vi "Calculate Vertex Array.vi"(8 "error in (no error)":errorcluster, 9 "Coordinates System":enum16{"Cartesian", "Cylindrical", "Spherical"}(ring)=enum."Spherical", 10 "3D Bar Datatype.lvclass in":refnum<class "3D Bar Datatype.lvclass">, 11 "Plot Representation In":T1) -> (0 "error out":errorcluster, 1 "Dup Coordinates System":enum16{"Cartesian", "Cylindrical", "Spherical"}(ring)=enum."Spherical", 2 "3D Bar Datatype.lvclass out":refnum<class "3D Bar Datatype.lvclass">, 3 "Plot Representation Out":T1)   [LabVIEW 2020, in "3D Bar Datatype.lvclass"]
uses:
  <vilib>/Math Plots/3D Math Plots/3D Bar/3D Bar Datatype/3D Bar Datatype.lvclass
  <vilib>/Math Plots/3D Math Plots/3D Plot/3D Plot/Typedef/Plot Representation.ctl
  <vilib>/Math Plots/3D Math Plots/3D Plot/3D Plot/Typedef/Range Clusters.ctl
  <vilib>/Math Plots/3D Math Plots/3D Plot/3D Plot/Typedef/Mesh Data.ctl
  <vilib>/Math Plots/3D Math Plots/3D Bar/3D Bar Datatype/3D Bar Datatype.lvclass/3D Bar Datatype.ctl
  <vilib>/Math Plots/3D Math Plots/3D Plot/3D Plot/3D Plot.lvclass
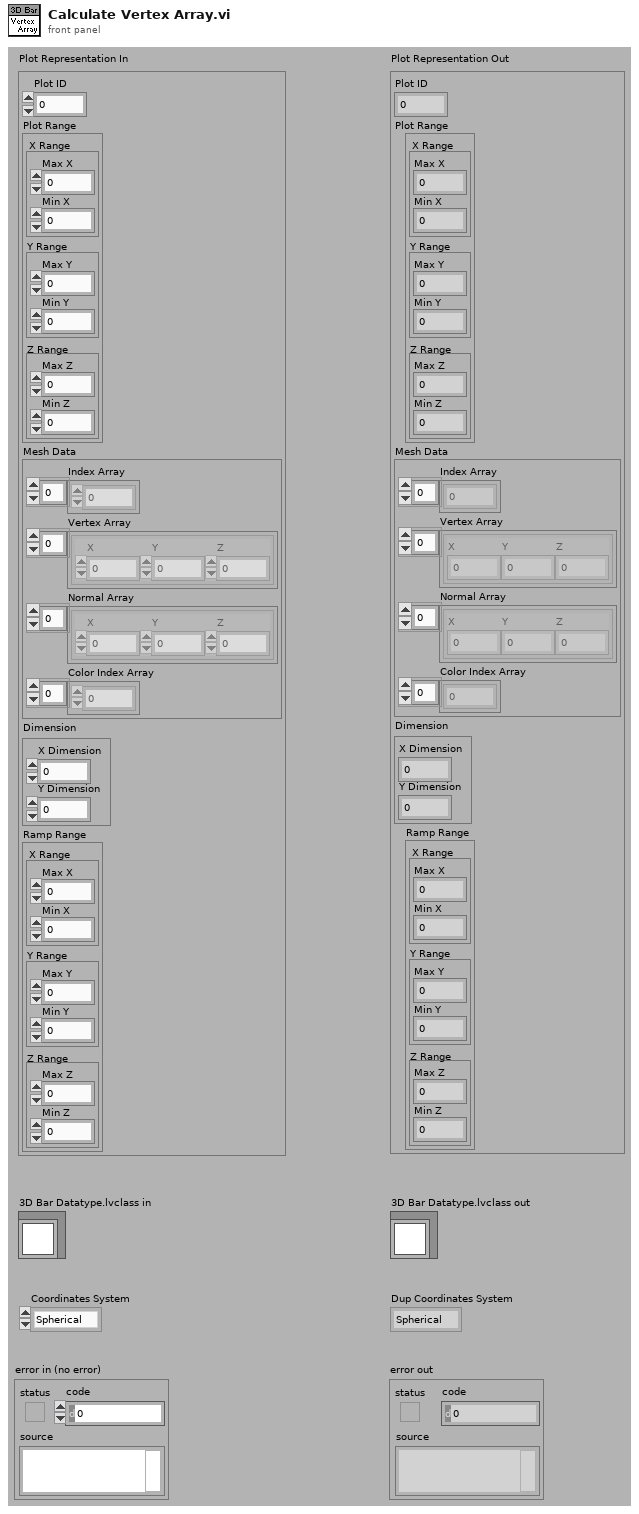
[diagram p1: front panel]
types:
  T1 = typedef "3D Plot.lvclass/Plot Representation.ctl" = cluster{"Plot ID":i32, "Plot Range":T2, "Mesh Data":T3, "Dimension":cluster{"X Dimension":i32, "Y Dimension":i32}, "Ramp Range":T2}
  T2 = typedef "3D Plot.lvclass/Range Clusters.ctl" = cluster{"X Range":cluster{"Max X":sgl, "Min X":sgl}, "Y Range":cluster{"Max Y":sgl, "Min Y":sgl}, "Z Range":cluster{"Max Z":sgl, "Min Z":sgl}}
  T3 = typedef "3D Plot.lvclass/Mesh Data.ctl" = cluster{"Index Array":u32[], "Vertex Array":cluster{"X":sgl, "Y":sgl, "Z":sgl}[], "Normal Array":cluster{"X":sgl, "Y":sgl, "Z":sgl}[], "Color Index Array":i32[]}
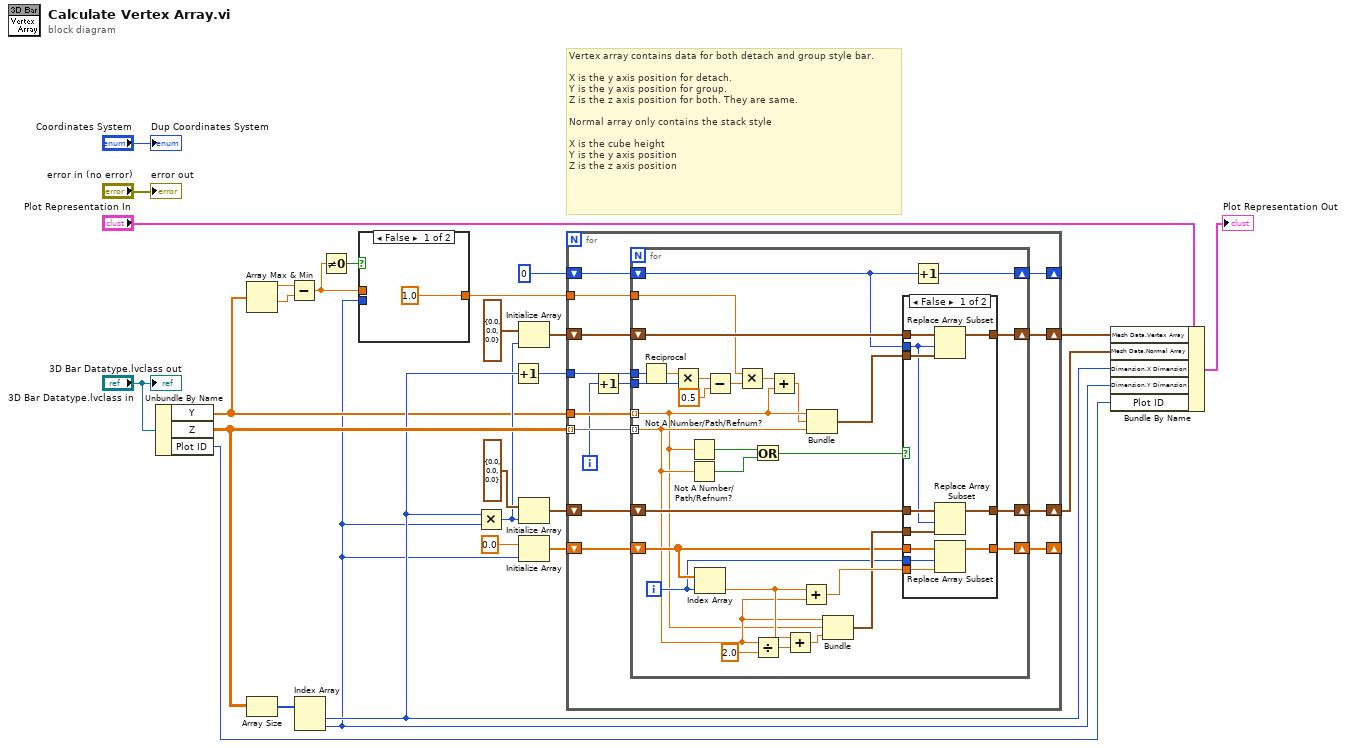
[diagram p0: block diagram]
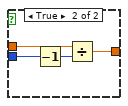
[diagram p2: hidden frame]
diagram:
  # "Vertex array contains data for both detach and group style bar. \n\nX is the y axis position for detach.\nY is the y axis position for group.\nZ is the z axis position for both. They are same.\n\nNormal array only contains the stack style\n\nX is the cube height\nY is the y axis position\nZ is the z axis position"
  n1 = Unbundle By Name("3D Bar Datatype.lvclass in") -> ("Y"=w7:sgl[], "Z"=w20:sgl[][], "Plot ID"=w19:i32)
  n2 = Array Max & Min(array=w7) -> (max value=w4:sgl, min value=w3:sgl)  [unwired: 2 out]
  n3 = Array Size(array=w20) -> (size(s)=w18:i32[])
  n4 = Subtract(x=w4, y=w3) -> (x-y=w2:sgl)
  n5 = Index Array(array=w18) -> (element #1=w15:i32, element #2=w5:i32)  [unwired: 2 in]
  n6 = Not Equal To 0?(x=w2) -> (x != 0?=w1:bool)
  n7 = case shown="False" w1 {
    tunnel: [sgl 1.0 w32] -> w6
    tunnel: w5 -> [_ w31]
    tunnel: w2 -> [_ w29]
    frame False {
    }
    frame True {
      n8 = Decrement(x=w31) -> (x-1=w30:i32)
      n9 = Divide(x=w29, y=w30) -> (x/y=w32:sgl)
    }
  }
  n10 = Multiply(x=w15, y=w5) -> (x*y=w11:i32)
  n11 = Increment(x=w15) -> (x+1=w21:i32)
  n12 = Initialize Array(cluster{"X":sgl, "Y":sgl, "Z":sgl} {"X"=0.0, "Y"=0.0, "Z"=0.0} ("3D Point"), w11) -> (w16:cluster{"X":sgl, "Y":sgl, "Z":sgl}[])
  n13 = Initialize Array(cluster{"X":sgl, "Y":sgl, "Z":sgl} {"X"=0.0, "Y"=0.0, "Z"=0.0} ("3D Point"), w11) -> (w10:cluster{"X":sgl, "Y":sgl, "Z":sgl}[])
  n14 = Initialize Array(sgl 0.0 ("y"), w5) -> (w9:sgl[])
  n15 = for {
    shift-right: [w45] -> w22
    shift-left: w16 -> [w46]
    tunnel: w20 -> [w44] mode=indexing
    tunnel: w7 -> [w43]
    tunnel: w21 -> [w42]
    shift-right: [w38] -> _
    shift-left: 0 -> [w39]
    shift-right: [w36] -> w8
    shift-left: w10 -> [w37]
    shift-right: [w34] -> _
    shift-left: w9 -> [w35]
    tunnel: w6 -> [w33]
    i -> [w41]
    n16 = Increment(x=w41) -> (x+1=w40:i32)
    n17 = for {
      shift-right: [w75] -> w45
      shift-left: w46 -> [w76]
      tunnel: w44 -> [w59] mode=indexing
      tunnel: w43 -> [w51] mode=indexing
      tunnel: w42 -> [w72]
      tunnel: w40 -> [w54]
      shift-right: [w73] -> w38
      shift-left: w39 -> [w63]
      shift-right: [w64] -> w36
      shift-left: w37 -> [w65]
      shift-right: [w61] -> w34
      shift-left: w35 -> [w62]
      tunnel: w33 -> [w48]
      i -> [w60]
      n18 = Reciprocal(x=w72) -> (1/x=w55:sgl)
      n19 = Multiply(x=w55, y=w54) -> (x*y=w53:sgl)
      n20 = Not A Number/Path/Refnum?(number/path/refnum=w51) -> (NaN/Path/Refnum?=w70:bool)
      n21 = Not A Number/Path/Refnum?(number/path/refnum=w59) -> (NaN/Path/Refnum?=w71:bool)
      n22 = Index Array(array=w62, index=w60) -> (element=w68:sgl)
      n23 = Subtract(x=w53, y=sgl 0.5) -> (x-y=w49:sgl)
      n24 = Multiply(x=w48, y=w49) -> (x*y=w47:sgl)
      n25 = Or(x=w70, y=w71) -> (x .or. y?=w56:bool)
      n26 = Divide(x=w59, y=sgl 2.0) -> (x/y=w58:sgl)
      n27 = Add(x=w47, y=w51) -> (x+y=w50:sgl)
      n28 = Add(x=w68, y=w58) -> (x+y=w67:sgl)
      n29 = Add(x=w68, y=w59) -> (x+y=w69:sgl)
      n30 = Bundle("Data"=w51, w50, "Data"=w59) -> (w74:cluster{"Data":sgl, sgl, "Data":sgl})  [unwired: 1 out]
      n31 = Bundle("Data"=w59, "Data"=w51, w67) -> (w66:cluster{"Data":sgl, "Data":sgl, sgl})  [unwired: 1 out]
      n32 = case shown="False" w56 {
        tunnel: w76 -> [w87 w90]
        tunnel: [w86 w90] -> w75
        tunnel: w74 -> [w85 _]
        tunnel: w69 -> [w84 _]
        tunnel: w66 -> [w83 _]
        tunnel: w65 -> [w82 w89]
        tunnel: [w81 w89] -> w64
        tunnel: w63 -> [w80 _]
        tunnel: w62 -> [w79 w88]
        tunnel: [w78 w88] -> w61
        tunnel: w60 -> [w77 _]
        frame False {
          n33 = Replace Array Subset(array=w87, new element=w85, index=w80) -> (w86:cluster{"X":sgl, "Y":sgl, "Z":sgl}[])
          n34 = Replace Array Subset(array=w82, new element=w83, index=w80) -> (w81:cluster{"X":sgl, "Y":sgl, "Z":sgl}[])
          n35 = Replace Array Subset(array=w79, new element=w84, index=w77) -> (w78:sgl[])
        }
        frame True {
        }
      }
      n36 = Increment(x=w63) -> (x+1=w73:i32)
    }
  }
  n37 = Bundle By Name(cluster="Plot Representation In", "Mesh Data.Vertex Array"=w22, "Mesh Data.Normal Array"=w8, "Dimension.X Dimension"=w15, "Dimension.Y Dimension"=w5, "Plot ID"=w19) -> (→"Plot Representation Out":T1)
  "error out" <- "error in (no error)"
  "3D Bar Datatype.lvclass out" <- "3D Bar Datatype.lvclass in"
  "Dup Coordinates System" <- "Coordinates System"
